vi "Handle Refresh Response.vi"(6 "Refresh Token":string, 8 "error in (no error)":errorcluster, 10 "Response Body":string, 11 "Async Authorization in":refnum<class "Async Authorization.lvclass">) -> (0 "error out":errorcluster, 3 "Asyn Authorization out":refnum<class "Async Authorization.lvclass">)   [LabVIEW 2020, in "OAuth2.lvlib" / "Async Authorization.lvclass"]
uses:
  Async Authorization.lvclass
  Async Authorization.lvclass/Async Authorization.ctl
  3b40fd08-d5a5-4162-adab-a042d9031a6d.vi
  <vilib>/Comparison/Equal/Equal Functor/Equal Functor.lvclass
  Authorization/Authorization.lvclass
  <vilib>/JDP Science/JSONtext/JSONtext.lvlib
  <vilib>/IlluminatedG/lv-web-crypto/lv-json/JSON/JSON.lvlib
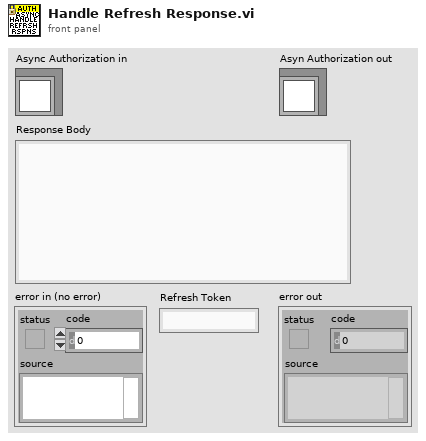
[diagram p1: front panel]
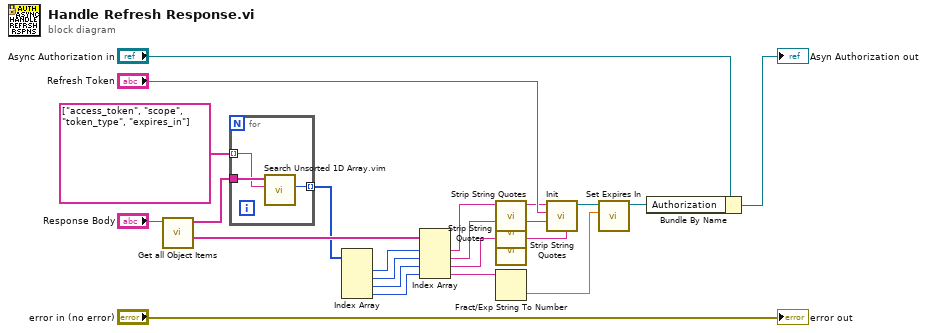
[diagram p0: block diagram]
diagram:
  n1 = call <vilib>:"Get all Object Items.vi"("JSON"="Response Body") -> ("<JSON>"=w14:string[], "Item Names"=w15:string[])  [unwired: 7 in, 2 out]
  n2 = for {
    tunnel: w15 -> [w26]
    tunnel: string[] ["access_token", "scope", "token_type", "expires_in"] ("Search Keys") -> [w25] mode=indexing
    tunnel: [w24] -> w12 mode=indexing
    n3 = call "Search Unsorted 1D Array.vim"("element"=w25, "unsorted 1D array"=w26) -> ("index of element"=w24:i32)  [unwired: 9 in]
  }
  n4 = Index Array(array=w12) -> (element #1=w8:i32, element #2=w11:i32, element #3=w10:i32, element #4=w9:i32)  [unwired: 4 in]
  n5 = Index Array(array=w14, index #1=w8, index #2=w11, index #3=w10, index #4=w9) -> (element #1=w5:string, element #2=w3:string, element #3=w1:string, element #4=w22:string)
  n6 = call <vilib>:"Strip String Quotes.vi"("JSON"=w5) -> ("Quotes Stripped"=w6:string)  [unwired: 10 in]
  n7 = call <vilib>:"Strip String Quotes.vi"("JSON"=w3) -> ("Quotes Stripped"=w4:string)  [unwired: 10 in]
  n8 = call <vilib>:"Strip String Quotes.vi"("JSON"=w1) -> ("Quotes Stripped"=w2:string)  [unwired: 10 in]
  n9 = Fract/Exp String To Number(string=w22) -> (number=w20:dbl)  [unwired: 3 in, 1 out]
  n10 = call "Init.vi"("Token Type"=w2, "Scope"=w4, "Refresh Token"="Refresh Token", "Access Token"=w6) -> ("Authorization"=w21:refnum<class "Authorization.lvclass">)  [unwired: 7 in]
  n11 = call "Set Expires In.vi"("Expires In"=w20, "Authorization in"=w21) -> ("Authorization out"=w19:refnum<class "Authorization.lvclass">)  [unwired: 9 in]
  n12 = Bundle By Name(cluster="Async Authorization in", "Authorization"=w19) -> (→"Asyn Authorization out":refnum<class "Async Authorization.lvclass">)
  "error out" <- "error in (no error)"
